vi "intakeStatus.vi"() -> ()   [LabVIEW 2016]
panel:
  out "intakeStatus":bool
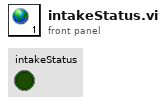
[diagram p1: front panel]
diagram:
